vi "Shut Down Device.vi"(8 "error in (no error)":errorcluster, 11 "Nikon Ti2 Stage in":refnum<class "Nikon Ti2 Stage.lvclass">) -> (0 "error out":errorcluster, 3 "Nikon Ti2 Stage out":refnum<class "Nikon Ti2 Stage.lvclass">)   [LabVIEW 2023, in "Nikon Ti2 Stage.lvlib" / "Nikon Ti2 Stage.lvclass"]
uses:
  Nikon Ti2 Stage.lvclass
  Nikon Ti2 Stage.lvclass/Nikon Ti2 Stage.ctl
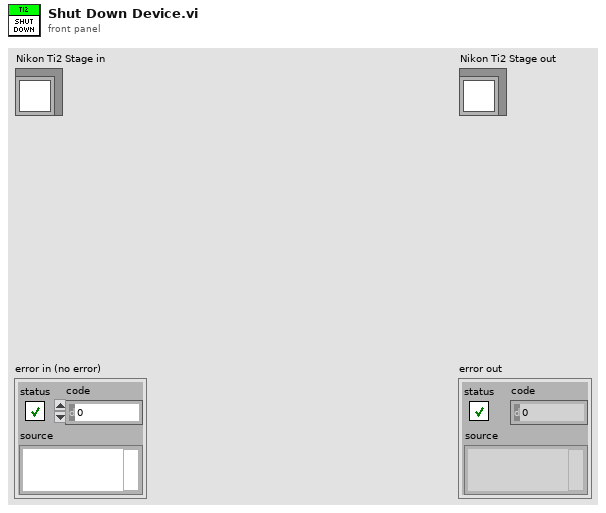
[diagram p1: front panel]
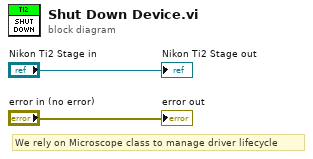
[diagram p0: block diagram]
diagram:
  # "We rely on Microscope class to manage driver lifecycle"
  "error out" <- "error in (no error)"
  "Nikon Ti2 Stage out" <- "Nikon Ti2 Stage in"
